vi "Test status global.vi"() -> ()   [LabVIEW 2014]
panel:
  in  "Test status":string
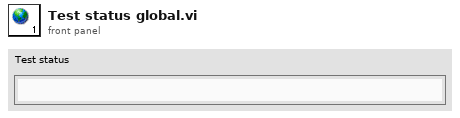
[diagram p1: front panel]
diagram:
